vi "check_set_ID_response.vi"(5 "RegEx parsing string in\n(\"(Rohde-Schwarz|Rohde&Schwarz|HAMEG),([^,]+)\")":string="(Rohde-Schwarz|Rohde&Schwarz|HAMEG),([^,]+)", 6 "Supported instruments in":string[](array[string]), 7 "Error if ID Query check fails":bool, 8 "error in":errorcluster, 9 "Aliases in (\"\")":string, 10 "IDN string in":string, 11 "VISA resource name":refnum<visa-resource-name>) -> (0 "error out":errorcluster, 1 "Instrument is supported":bool, 2 "Instrument type out":string, 3 "VISA resource name out":refnum<visa-resource-name>)   [LabVIEW 2014, in "rszvl_rsidr_core.lvlib"]
uses:
  rszvl_rsidr_core.lvlib
  type_Error_Codes.ctl
  Match Regular Expression.xnode
panel:
  out "Alias is used":bool
  # "Aliases expression can be used\nfor mapping purposes. Syntax:\n<physical device1_Regex> -> <alias1>\\n\n<physical device2_Regex> -> <alias2>\\n\n\nExamples:\nto have FSWP-33 to be treated as FSVR:\n^FSWP-33$ -> FSVR\nany FSVA to be treated as FSV:\n^FSVA-[0-9]+$ -> FSV"
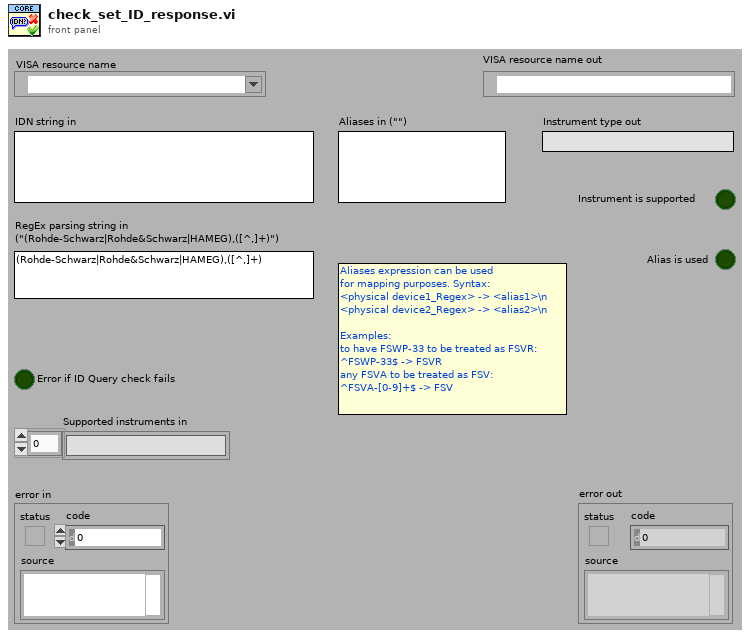
[diagram p1: front panel]
types:
  T1 = enum16{"Initialize", "GetData", "SetData", "Clear"}
  T2 = typedef "rszvl_rsidr_core.lvlib/type_Error_Codes.ctl" = enum16{"No_error", "VISA_err_ResourceNotFound", "VISA_err_Timeout", "VISA_warn_MoreDataAvailable", "RS_err_MissingCallback", "RS_err_InvalidAttribute", "RS_err_InvalidValue", "RS_err_UnknownResource", "RS_err_AlreadyInitialized", "RS_err_InstrumentStatus", "RS_err_BadRepCapName", "RS_err_TypesMismatch", "RS_err_ValueNotSupported", "RS_err_InvalidRngTable", "RS_err_IDqueryFail", "RS_err_UnexpResponse", "VISA_warn_ConfigNotLoaded", "RS_err_AttributeNotReadable", "RS_err_AttributeNotWritable", "RS_err_InstrumentType", "RS_err_InstrumentOption", "VISA_err_InvalidSize", "RS_err_ReliabilityIndicator", "VISA_warn_UnknownStatus", "VISA_warn_TermCharRead", "VISA_err_IO_error"}
  T3 = typedef "rszvl_rsidr_core.lvlib/type_Session_Data.ctl" = cluster{"Instr type":string, "Instr type for err. msg.":string, "Installed Options":string[], "OPC Timeout":i32, "Query Instrument Status":bool, "Check Range":bool, "Check Options":bool, "Add LF to Write":bool, "Simulate":bool, "Logging":bool, "Logging params":variant, "Interface Type":enum16{"Unknown", "GPIB", "VXI", "GPIB_VXI", "ASRL", "PXI", "TCPIP", "USB", "SOCKET"}, "Fast Sweep":i32, "AdditionalFlags":i32, "WaitBeforeWrite":i32, "WaitBeforeRead":i32, "BinDataChunkSize":i64}
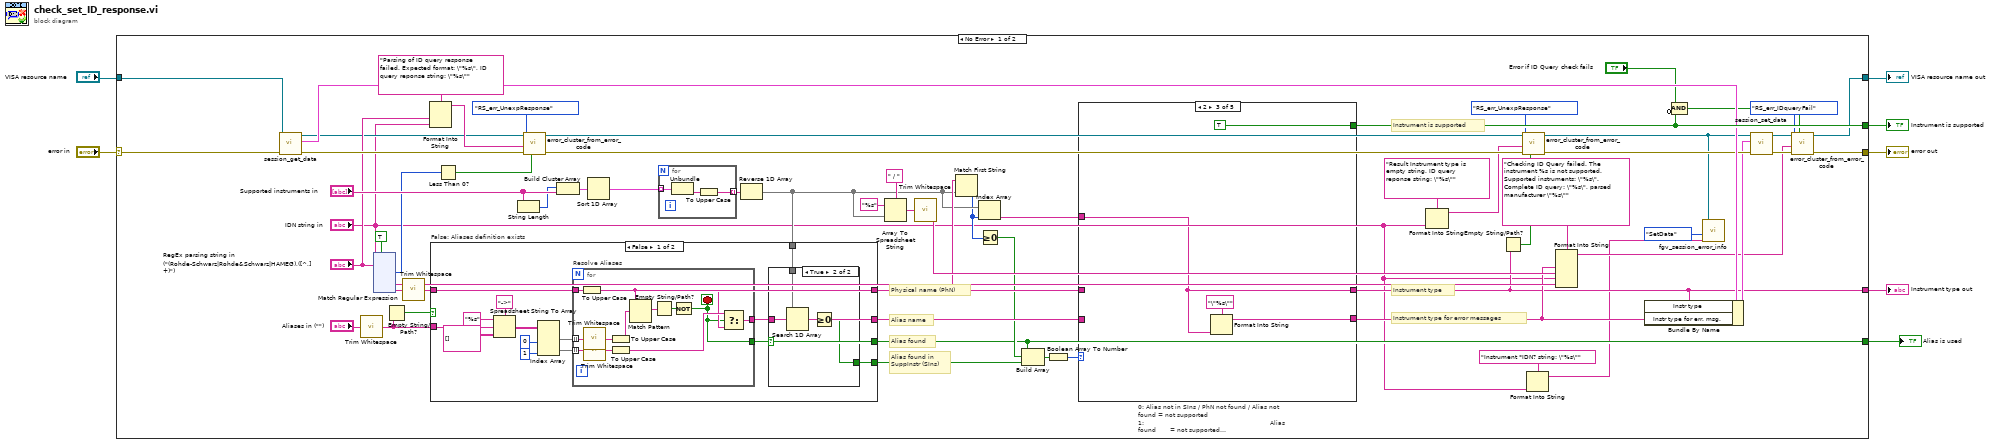
[diagram p0: block diagram]
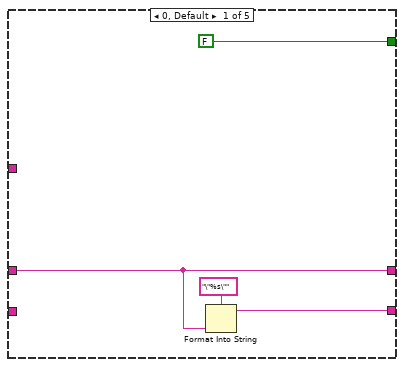
[diagram p4: hidden frame]
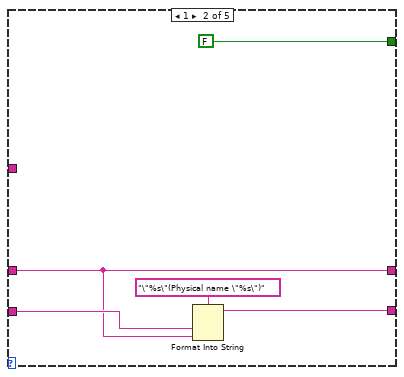
[diagram p5: hidden frame]
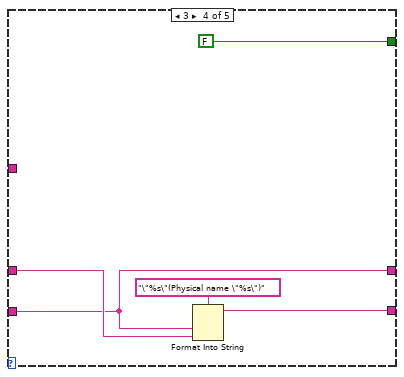
[diagram p6: hidden frame]
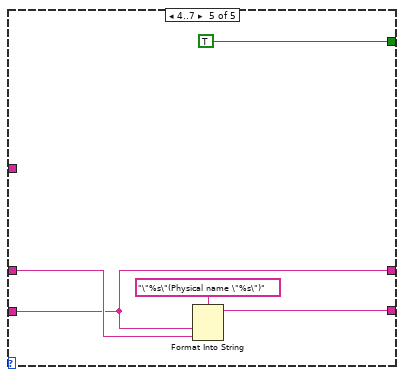
[diagram p7: hidden frame]
diagram:
  n1 = case shown="No Error" "error in" {
    selector: "error in" -> [w67 w242]
    tunnel: [w69 w242] -> w7
    tunnel: [w36 _] -> w5
    tunnel: [w68 _] -> w4
    tunnel: "VISA resource name" -> [w65 w241]
    tunnel: [w28 w241] -> w2
    tunnel: [w13 _] -> w1
    frame No Error {
      # "Alias found in\nSuppInstr (SIns)"
      # "Alias found"
      # "Instrument is supported"
      # "Instrument type for error messages"
      # "Instrument type"
      # "Physical name (PhN)"
      # "Alias name"
      n2 = call "session_get_data.vi"("error in"=w67, "VISA resource name"=w65) -> ("error out"=w66:errorcluster, "Session User Data out"=w64:T3, "VISA resource name out"=w32:refnum<visa-resource-name>)  [unwired: 7 in]
      n3 = call "Trim Whitespace.vi"("string"="Aliases in (\"\")") -> ("trimmed string"=w50:string)  [unwired: 1 in]
      n4 = xnode ("Match Regular Expression")("input string"="IDN string in", "regular expression"="RegEx parsing string in\n(\"(Rohde-Schwarz|Rohde&Schwarz|HAMEG),([^,]+)\")", "ignore case? (F)"=TRUE) -> ("offset past match"=w48:i32, "submatch 1"=w54:string, "submatch 2"=w18:string)  [unwired: 3 in, 4 out]
      n5 = Empty String/Path?(string/path=w50) -> (empty?=w49:bool)
      n6 = call "Trim Whitespace.vi"("string"=w18) -> ("trimmed string"=w17:string)  [unwired: 1 in]
      n7 = Format Into String(format string="Parsing of ID query response failed. Expected format: \"%s\", ID query reponse string: \"%s\"", "RegEx parsing string in\n(\"(Rohde-Schwarz|Rohde&Schwarz|HAMEG),([^,]+)\")", "IDN string in") -> (resulting string=w34:string)  [unwired: 2 in, 1 out]
      n8 = Less Than 0?(x=w48) -> (x < 0?=w47:bool)
      n9 = String Length(string="Supported instruments in") -> (length=w51:i32[])
      n10 = call "error_cluster_from_error_code.vi"("error creation enabled (T)"=w47, "error in"=w66, "error message (\"\")"=w34, "Error Enum in"=type_Error_Codes."RS_err_UnexpResponse", "VISA resource name"=w32) -> ("error out"=w44:errorcluster, "VISA resource name out"=w33:refnum<visa-resource-name>)  [unwired: 5 in]
      n11 = Build Cluster Array ("Index & Bundle Cluster Array")(w51, "Supported instruments in") -> (w56:cluster{"String":i32, "String":string}[])
      n12 = Sort 1D Array(array=w56) -> (sorted array=w55:cluster{"String":i32, "String":string}[])
      n13 = for {
        tunnel: w55 -> [w103] mode=indexing
        tunnel: [w101] -> w35 mode=indexing
        n14 = Unbundle(w103) -> ("String"=w102:string)  [unwired: 1 out]
        n15 = To Upper Case(1:w102) -> (0:w101:string)
      }
      n16 = Reverse 1D Array(array=w35) -> (reversed array=w20:string[])
      n17 = case "False: Aliases definition exists" shown="False" w49 {
        tunnel: w17 -> [w70 w100]
        tunnel: [w72 _] -> w58
        tunnel: [w74 _] -> w13
        tunnel: w50 -> [w78 _]
        tunnel: [w70 w100] -> w21
        tunnel: w20 -> [w73 _]
        tunnel: [w71 _] -> w15
        frame False {
          n18 = Spreadsheet String To Array(delimiter (Tab)="->", format string="%s", spreadsheet string=w78, array type (2D Dbl)=string[][] [] ("Array")) -> (array=w80:string[][])
          n19 = Index Array(array=w80, index (col) #1=0 ("index (row)"), index (col) #2=1 ("index (row)")) -> (element #1=w75:string[], element #2=w79:string[])  [unwired: 2 in]
          n20 = for "Resolve Aliases" {
            tunnel: w75 -> [w99] mode=indexing
            tunnel: w79 -> [w97] mode=indexing
            tunnel: [w95] -> w72
            tunnel: [w88] -> w74
            tunnel: w70 -> [w93]
            stop <- w88 stop-if-true
            n21 = To Upper Case(1:w93) -> (0:w92:string)
            n22 = call "Trim Whitespace.vi"("string"=w99) -> ("trimmed string"=w98:string)  [unwired: 1 in]
            n23 = call "Trim Whitespace.vi"("string"=w97) -> ("trimmed string"=w96:string)  [unwired: 1 in]
            n24 = To Upper Case(1:w98) -> (0:w91:string)
            n25 = To Upper Case(1:w96) -> (0:w94:string)
            n26 = Match Pattern(string=w92, regular expression=w91) -> (match substring=w90:string)  [unwired: 1 in, 3 out]
            n27 = Empty String/Path?(string/path=w90) -> (empty?=w89:bool)
            n28 = Not(x=w89) -> (.not. x?=w88:bool)
            n29 = Select(t=w94, s=w88, f=w92) -> (s? t:f=w95:string)
          }
          n30 = case shown="True" w74 {
            tunnel: w73 -> [_ w87]
            tunnel: w72 -> [_ w86]
            tunnel: [_ w84] -> w71
            frame False {
            }
            frame True {
              n31 = Search 1D Array(1D array=w87, element=w86) -> (index of element=w85:i32)  [unwired: 1 in]
              n32 = Greater Or Equal To 0?(x=w85) -> (x >= 0?=w84:bool)
            }
          }
        }
        frame True {
        }
      }
      n33 = Array To Spreadsheet String(delimiter (Tab)=" / ", array=w20, 3:"%s" ("format string")) -> (spreadsheet string=w61:string)
      n34 = call "Trim Whitespace.vi"("string"=w61) -> ("trimmed string"=w42:string)  [unwired: 1 in]
      n35 = Match First String(2:w20, 3:w21) -> (0:w19:i32)  [unwired: 1 out]
      n36 = Index Array(array=w20, index=w19) -> (element=w14:string)
      n37 = Greater Or Equal To 0?(x=w19) -> (x >= 0?=w16:bool)
      n38 = Build Array(w13, w16, w15) -> (w23:bool[])
      n39 = Boolean Array To Number(Boolean array=w23) -> (number=w22:u32)
      n40 = case "0: Alias not in SIns / PhN not found / Alias not found = not supported\n1:                                                               Alias found       = not supported\n2:                                 PhN found                                      = supported PhN\n3: Alias not in SIns    PhN found           Alias found       = not supported\n4..7: Alias in SIns                                                                 = supported allias" shown="2" w22 {
        tunnel: w58 -> [_ w109 _ w117 w122]
        tunnel: w21 -> [w105 w108 _ w118 w123]
        tunnel: [w105 w108 w113 w117 w122] -> w36
        tunnel: [w104 w110 w114 w119 w124] -> w39
        tunnel: [FALSE FALSE TRUE FALSE TRUE] -> w68
        tunnel: w14 -> [_ _ w113 _ _]
        frame 0, Default {
          n41 = Format Into String(format string="\"%s\"", w105) -> (resulting string=w104:string)  [unwired: 2 in, 1 out]
        }
        frame 1 {
          n42 = Format Into String(format string="\"%s\"(Physical name \"%s\")", w109, w108) -> (resulting string=w110:string)  [unwired: 2 in, 1 out]
        }
        frame 2 {
          n43 = Format Into String(format string="\"%s\"", w113) -> (resulting string=w114:string)  [unwired: 2 in, 1 out]
        }
        frame 3 {
          n44 = Format Into String(format string="\"%s\"(Physical name \"%s\")", w117, w118) -> (resulting string=w119:string)  [unwired: 2 in, 1 out]
        }
        frame 4..7 {
          n45 = Format Into String(format string="\"%s\"(Physical name \"%s\")", w122, w123) -> (resulting string=w124:string)  [unwired: 2 in, 1 out]
        }
      }
      n46 = Format Into String(format string="Result Instrument type is empty string. ID query reponse string: \"%s\"", "IDN string in") -> (resulting string=w31:string)  [unwired: 2 in, 1 out]
      n47 = Empty String/Path?(string/path=w36) -> (empty?=w43:bool)
      n48 = call "error_cluster_from_error_code.vi"("error creation enabled (T)"=w43, "error in"=w44, "error message (\"\")"=w31, "Error Enum in"=type_Error_Codes."RS_err_UnexpResponse", "VISA resource name"=w33) -> ("error out"=w38:errorcluster, "VISA resource name out"=w11:refnum<visa-resource-name>)  [unwired: 5 in]
      n49 = Format Into String(format string="Instrument *IDN? string: \"%s\"", "IDN string in") -> (resulting string=w9:string)  [unwired: 2 in, 1 out]
      n50 = Format Into String(format string="Checking ID Query failed. The instrument %s is not supported. Supported instruments: \"%s\". Complete ID query: \"%s\", parsed manufacturer \"%s\"", w39, w42, "IDN string in", w54) -> (resulting string=w27:string)  [unwired: 2 in, 1 out]
      n51 = Bundle By Name(cluster=w64, "Instr type"=w36, "Instr type for err. msg."=w39) -> (w37:T3)
      n52 = Compound Arithmetic op=AND("Error if ID Query check fails", invert w68) -> (w52:bool)
      n53 = call "fgv_session_error_info.vi"("Session Error Info in (\"\")"=w9, "Operation"=T1."SetData", "Session in"=w11) -> ()  [unwired: 4 in, 1 out]
      n54 = call "session_set_data.vi"("error in"=w38, "Session User Data in"=w37, "VISA resource name"=w11) -> ("error out"=w40:errorcluster, "VISA resource name out"=w29:refnum<visa-resource-name>)  [unwired: 7 in]
      n55 = call "error_cluster_from_error_code.vi"("error creation enabled (T)"=w52, "error in"=w40, "error message (\"\")"=w27, "Error Enum in"=type_Error_Codes."RS_err_IDqueryFail", "VISA resource name"=w29) -> ("error out"=w69:errorcluster, "VISA resource name out"=w28:refnum<visa-resource-name>)  [unwired: 5 in]
    }
    frame Error {
    }
  }
  "VISA resource name out" <- w2
  "error out" <- w7
  "Instrument type out" <- w5
  "Instrument is supported" <- w4
  "Alias is used" <- w1
